vi "HIPOT-GPT9803 IR TEST.vi"() -> ()   [LabVIEW 2021]
uses:
  LVdriver_GPT-9800_GSB_2011_V1_E/GPT-9800_GSB_L2011/GPT-9000.lvlib
panel:
  out "RESULT":bool
  out "error out":errorcluster
  out "Error Message":string
  out "Time":string
  out "Impedance":string
  out "Voltage":string
  out "VISA resource name out":refnum<visa-resource-name>
  in  "error in":errorcluster
  in  "IR Test Time(S)":sgl=1.0 min=1 max=999.9 format="%.1f"
  in  "Ramp Time":sgl=1.0 min=0.1 max=999.9 format="%.1f"
  in  "IR voltage(kV)":sgl=0.1 min=0.0499 max=1.0001 step=0.05 format="%.2f"
  in  "Configure RS232 Baud Rate":u32(ring)=115200 items=["9600"=9600, "19200"=19200, "38400"=38400, "57600"=57600, "115200"=115200]
  in  "VISA resource name":refnum<visa-resource-name>
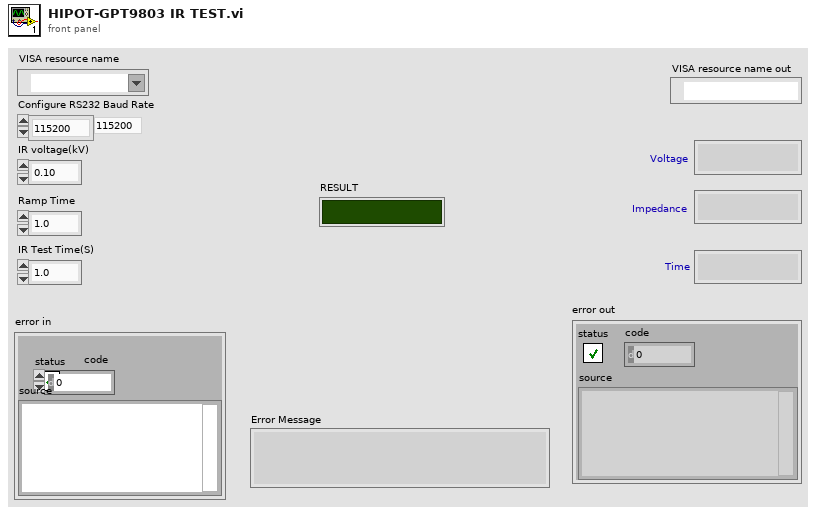
[diagram p1: front panel]
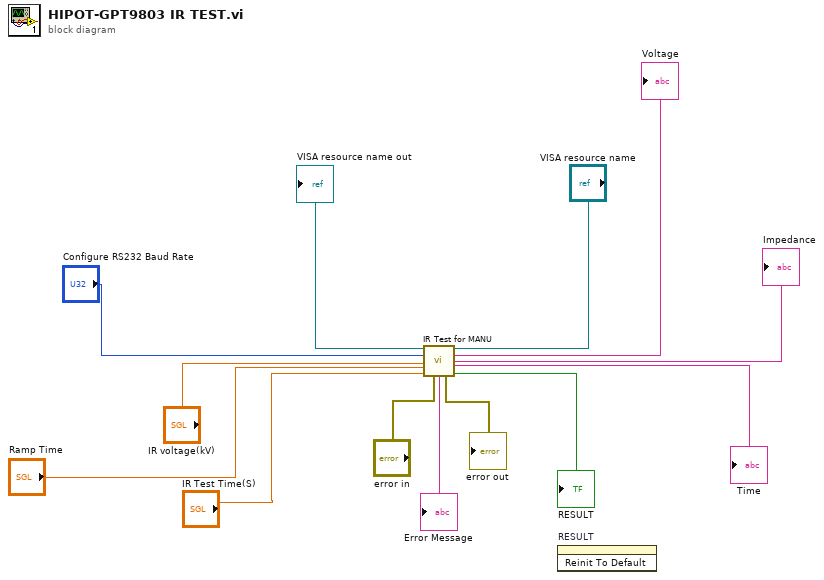
[diagram p0: block diagram]
diagram:
  n1 = call "IR Test for MANU.vi"("VISA resource name"="VISA resource name", "Configure RS232 Baud Rate"="Configure RS232 Baud Rate", "IR voltage(kV)"="IR voltage(kV)", "Ramp Time"="Ramp Time", "IR Test Time(S)"="IR Test Time(S)", "error in"="error in") -> ("VISA resource name out"=→"VISA resource name out":refnum<visa-resource-name>, "Voltage"=→"Voltage":string, "Impedance"=→"Impedance":string, "Time"=→"Time":string, "Error Message"=→"Error Message":string, "error out"=→"error out":errorcluster, "RESULT"=→"RESULT":bool)  [unwired: 3 in]
  n2 = invoke on="RESULT" class="Bool (strict)" method="Reinit To Default"() -> ()  [unwired: 3 in, 3 out]
